vi "make_axes_ticks.vi"(7 "Ticks Properties":T1, 8 "length":sgl, 11 "Scene Object In":refnum<vi>) -> (3 "Scene Object Out":refnum<vi>)   [LabVIEW 2020, in "3DPC_SurfacePlot.xctl"]
uses:
  <vilib>/Native 3D Graph/xcontrol/3DPC_SurfacePlot.xctl
  <vilib>/Native 3D Graph/typedefs/prop_axes_ticks.ctl
  <vilib>/picture/3D Picture Control/Object/Create Object (name).vi
  <vilib>/picture/3D Picture Control/NI_3D Picture Control.lvlib
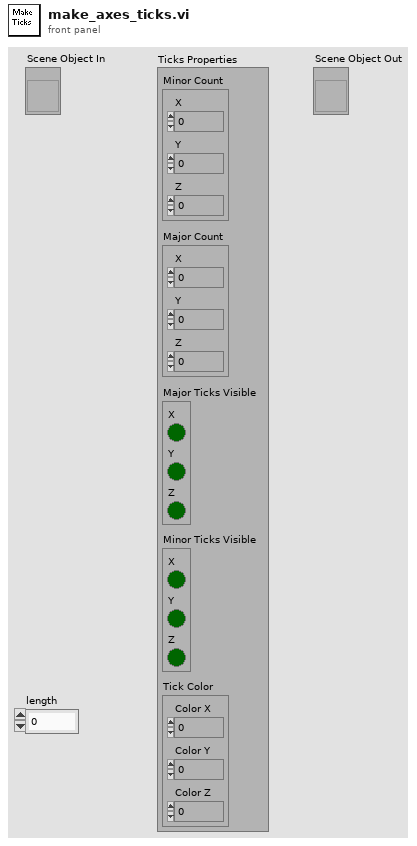
[diagram p1: front panel]
types:
  T1 = typedef "3DPC_SurfacePlot.xctl/prop_axes_ticks.ctl" = cluster{"Minor Count":cluster{"X":i32, "Y":i32, "Z":i32}, "Major Count":cluster{"X":i32, "Y":i32, "Z":i32}, "Major Ticks Visible":cluster{"X":bool, "Y":bool, "Z":bool}, "Minor Ticks Visible":cluster{"X":bool, "Y":bool, "Z":bool}, "Tick Color":cluster{"Color X":u32, "Color Y":u32, "Color Z":u32}}
  T2 = cluster{"Color X":u32, "Color Y":u32, "Color Z":u32}
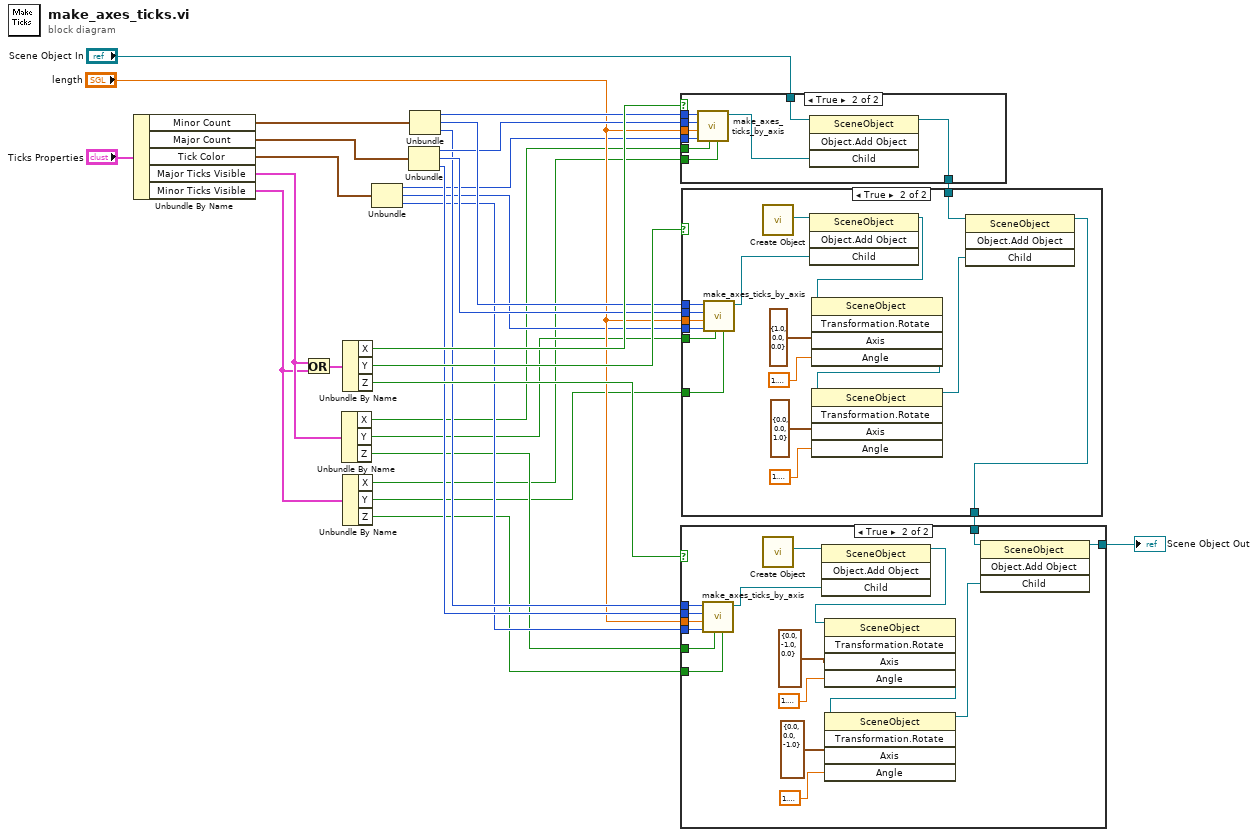
[diagram p0: block diagram]
diagram:
  n1 = Unbundle By Name("Ticks Properties") -> ("Minor Count"=w25:cluster{"X":i32, "Y":i32, "Z":i32}, "Major Count"=w24:cluster{"X":i32, "Y":i32, "Z":i32}, "Tick Color"=w13:T2, "Major Ticks Visible"=w8:cluster{"X":bool, "Y":bool, "Z":bool}, "Minor Ticks Visible"=w7:cluster{"X":bool, "Y":bool, "Z":bool})
  n2 = Or(x=w8, y=w7) -> (x .or. y?=w9:cluster{"X":bool, "Y":bool, "Z":bool})
  n3 = Unbundle By Name(w8) -> ("X"=w6:bool, "Y"=w5:bool, "Z"=w4:bool)
  n4 = Unbundle By Name(w9) -> ("X"=w23:bool, "Y"=w22:bool, "Z"=w21:bool)
  n5 = Unbundle By Name(w7) -> ("X"=w3:bool, "Y"=w2:bool, "Z"=w1:bool)
  n6 = Unbundle(w13) -> ("Color X"=w12:u32, "Color Y"=w11:u32, "Color Z"=w10:u32)
  n7 = Unbundle(w24) -> ("X"=w17:i32, "Y"=w19:i32, "Z"=w15:i32)
  n8 = Unbundle(w25) -> ("X"=w18:i32, "Y"=w20:i32, "Z"=w16:i32)
  n9 = case shown="True" w23 {
    tunnel: "Scene Object In" -> [w31 w40]
    tunnel: [w31 w39] -> w29
    tunnel: w18 -> [_ w37]
    tunnel: w17 -> [_ w36]
    tunnel: "length" -> [_ w35]
    tunnel: w12 -> [_ w34]
    tunnel: w6 -> [_ w33]
    tunnel: w3 -> [_ w32]
    frame False {
    }
    frame True {
      n10 = call <vilib>:"make_axes_ticks_by_axis.vi"("Draw Minor"=w32, "Draw Major"=w33, "Color"=w34, "length"=w35, "major ticks"=w36, "minor ticks"=w37) -> ("Scene:New Object"=w38:refnum<vi>)  [unwired: 1 in, 4 out]
      n11 = invoke class="SceneObject" method="Object.Add Object"(reference=w40, "Child"=w38) -> (reference out=w39:refnum<vi>)  [unwired: 2 in, 3 out]
    }
  }
  n12 = case shown="True" w22 {
    tunnel: w29 -> [w41 w57]
    tunnel: [w41 w56] -> w28
    tunnel: w20 -> [_ w47]
    tunnel: w19 -> [_ w46]
    tunnel: "length" -> [_ w45]
    tunnel: w11 -> [_ w44]
    tunnel: w5 -> [_ w43]
    tunnel: w2 -> [_ w42]
    frame False {
    }
    frame True {
      n13 = call <vilib>:"make_axes_ticks_by_axis.vi"("Draw Minor"=w42, "Draw Major"=w43, "Color"=w44, "length"=w45, "major ticks"=w46, "minor ticks"=w47) -> ("Scene:New Object"=w48:refnum<vi>)  [unwired: 1 in, 4 out]
      n14 = call-poly <vilib>:"Create Object.vi"() -> ("Scene:New Object"=w58:refnum<vi>)  [unwired: 10 in, 1 out]
      n15 = invoke class="SceneObject" method="Object.Add Object"(reference=w58, "Child"=w48) -> (reference out=w55:refnum<vi>)  [unwired: 2 in, 3 out]
      n16 = invoke class="SceneObject" method="Transformation.Rotate"(reference=w55, "Axis"=cluster{"X":sgl, "Y":sgl, "Z":sgl} {"X"=1.0, "Y"=0.0, "Z"=0.0}, "Angle"=1.5707963267948966) -> (reference out=w54:refnum<vi>)  [unwired: 2 in, 4 out]
      n17 = invoke class="SceneObject" method="Transformation.Rotate"(reference=w54, "Axis"=cluster{"X":sgl, "Y":sgl, "Z":sgl} {"X"=0.0, "Y"=0.0, "Z"=1.0}, "Angle"=1.5707963267948966) -> (reference out=w53:refnum<vi>)  [unwired: 2 in, 4 out]
      n18 = invoke class="SceneObject" method="Object.Add Object"(reference=w57, "Child"=w53) -> (reference out=w56:refnum<vi>)  [unwired: 2 in, 3 out]
    }
  }
  n19 = case shown="True" w21 {
    tunnel: w28 -> [w59 w75]
    tunnel: [w59 w74] -> w27
    tunnel: w16 -> [_ w66]
    tunnel: w15 -> [_ w65]
    tunnel: "length" -> [_ w64]
    tunnel: w10 -> [_ w63]
    tunnel: w4 -> [_ w61]
    tunnel: w1 -> [_ w60]
    frame False {
    }
    frame True {
      n20 = call <vilib>:"make_axes_ticks_by_axis.vi"("Draw Minor"=w60, "Draw Major"=w61, "Color"=w63, "length"=w64, "major ticks"=w65, "minor ticks"=w66) -> ("Scene:New Object"=w62:refnum<vi>)  [unwired: 1 in, 4 out]
      n21 = call-poly <vilib>:"Create Object.vi"() -> ("Scene:New Object"=w76:refnum<vi>)  [unwired: 10 in, 1 out]
      n22 = invoke class="SceneObject" method="Object.Add Object"(reference=w76, "Child"=w62) -> (reference out=w73:refnum<vi>)  [unwired: 2 in, 3 out]
      n23 = invoke class="SceneObject" method="Transformation.Rotate"(reference=w73, "Axis"=cluster{"X":sgl, "Y":sgl, "Z":sgl} {"X"=0.0, "Y"=-1.0, "Z"=0.0}, "Angle"=1.5707963267948966) -> (reference out=w72:refnum<vi>)  [unwired: 2 in, 4 out]
      n24 = invoke class="SceneObject" method="Transformation.Rotate"(reference=w72, "Axis"=cluster{"X":sgl, "Y":sgl, "Z":sgl} {"X"=0.0, "Y"=0.0, "Z"=-1.0}, "Angle"=1.5707963267948966) -> (reference out=w71:refnum<vi>)  [unwired: 2 in, 4 out]
      n25 = invoke class="SceneObject" method="Object.Add Object"(reference=w75, "Child"=w71) -> (reference out=w74:refnum<vi>)  [unwired: 2 in, 3 out]
    }
  }
  "Scene Object Out" <- w27
